vi "Arrays_Size to same.vi"(6 "Primary Default In":variant, 7 "Secondary Default In":variant, 8 "Select In":T1, 9 "Primary Array In":variant[](array[variant]), 11 "Secondary Array In":variant[](array[variant])) -> (1 "Primary Array Out":variant[](array[variant]), 3 "Secondary Array Out":variant[](array[variant]))   [LabVIEW 2015]
uses:
  TypeDefs_Utility/ENUM_Array_Size type select.ctl
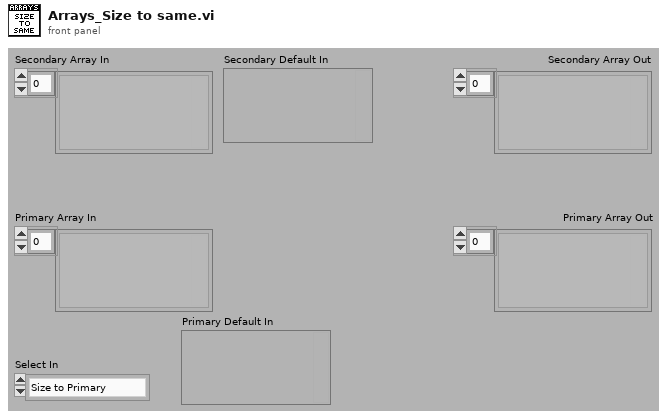
[diagram p1: front panel]
types:
  T1 = typedef "ENUM_Array_Size type select.ctl" = enum16{"Size to Primary", "Size to Secondary", "Size to Largest", "Size to Smallest"}
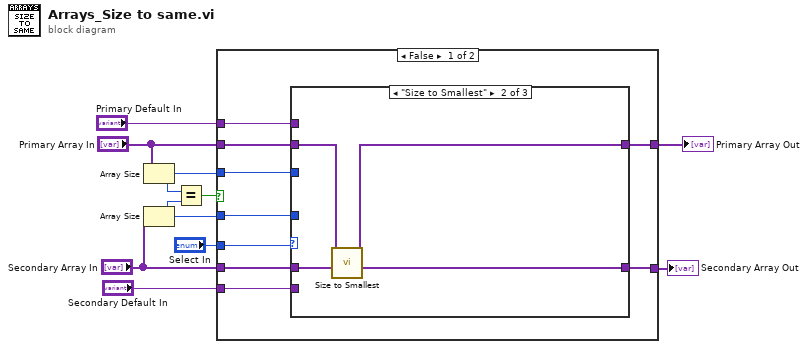
[diagram p0: block diagram]
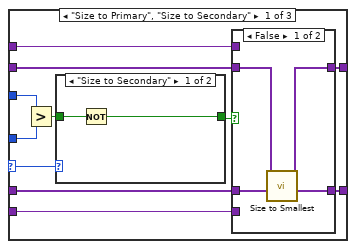
[diagram p2: hidden frame]
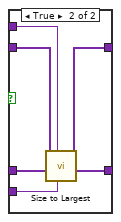
[diagram p3: hidden frame]
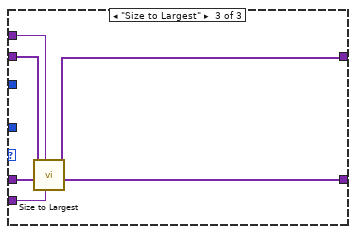
[diagram p5: hidden frame]
diagram:
  n1 = Array Size(array="Primary Array In") -> (size(s)=w5:i32)
  n2 = Array Size(array="Secondary Array In") -> (size(s)=w4:i32)
  n3 = Equal?(x=w5, y=w4) -> (x = y?=w10:bool)
  n4 = case shown="False" w10 {
    tunnel: "Secondary Array In" -> [w17 w55]
    tunnel: [w14 w55] -> w8
    tunnel: "Primary Array In" -> [w16 w54]
    tunnel: [w13 w54] -> w6
    tunnel: w5 -> [w12 _]
    tunnel: w4 -> [w11 _]
    tunnel: "Primary Default In" -> [w15 _]
    tunnel: "Secondary Default In" -> [w18 _]
    tunnel: "Select In" -> [w19 _]
    frame False {
      n5 = case shown="\"Size to Smallest\"" w19 {
        selector: w19 -> [w30 _ _]
        tunnel: w18 -> [w23 _ w50]
        tunnel: w17 -> [w25 w47 w51]
        tunnel: w16 -> [w21 w45 w53]
        tunnel: w15 -> [w22 _ w52]
        tunnel: [w24 w46 w49] -> w14
        tunnel: [w20 w44 w48] -> w13
        tunnel: w12 -> [w29 _ _]
        tunnel: w11 -> [w28 _ _]
        frame "Size to Primary", "Size to Secondary" {
          n6 = Greater?(x=w29, y=w28) -> (0:w27:bool)
          n7 = case shown="\"Size to Secondary\"" w30 {
            tunnel: w27 -> [w42 w43]
            tunnel: [w41 w43] -> w26
            frame "Size to Secondary" {
              n8 = Not(x=w42) -> (.not. x?=w41:bool)
            }
            frame "Size to Primary", Default {
            }
          }
          n9 = case shown="False" w26 {
            tunnel: w25 -> [w34 w40]
            tunnel: [w33 w39] -> w24
            tunnel: w23 -> [_ w38]
            tunnel: w22 -> [_ w37]
            tunnel: w21 -> [w32 w36]
            tunnel: [w31 w35] -> w20
            frame False {
              n10 = call "Size to Smallest.vi"("Secondary Array In"=w34, "Primary Array In"=w32) -> ("Secondary Array Out"=w33:variant[], "Primary Array Out"=w31:variant[])  [unwired: 8 in]
            }
            frame True {
              n11 = call "Size to Largest.vi"("Secondary Default In"=w38, "Primary Default In"=w37, "Secondary Array In"=w40, "Primary Array In"=w36) -> ("Secondary Array Out"=w39:variant[], "Primary Array Out"=w35:variant[])  [unwired: 6 in]
            }
          }
        }
        frame "Size to Smallest" {
          n12 = call "Size to Smallest.vi"("Secondary Array In"=w47, "Primary Array In"=w45) -> ("Secondary Array Out"=w46:variant[], "Primary Array Out"=w44:variant[])  [unwired: 8 in]
        }
        frame "Size to Largest" {
          n13 = call "Size to Largest.vi"("Secondary Default In"=w50, "Primary Default In"=w52, "Secondary Array In"=w51, "Primary Array In"=w53) -> ("Secondary Array Out"=w49:variant[], "Primary Array Out"=w48:variant[])  [unwired: 6 in]
        }
      }
    }
    frame True {
    }
  }
  "Secondary Array Out" <- w8
  "Primary Array Out" <- w6
